vi "esm_Set Target CPU Monitoring__NATIONAL INSTRUMENTS.vi"(8 "error in (no error)":errorcluster, 10 "CPU Monitoring On":bool=TRUE, 11 "application reference":refnum<vi>) -> (0 "error out":errorcluster, 3 "application reference out":refnum<vi>)   [LabVIEW 2010, in "kevLib2010.lvlib"]
uses:
  kevLib2010.lvlib
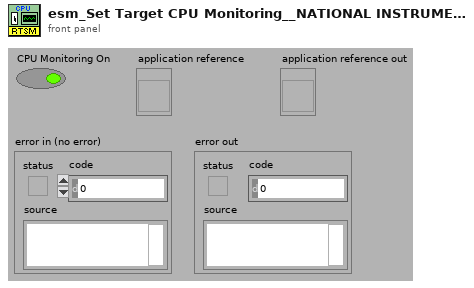
[diagram p1: front panel]
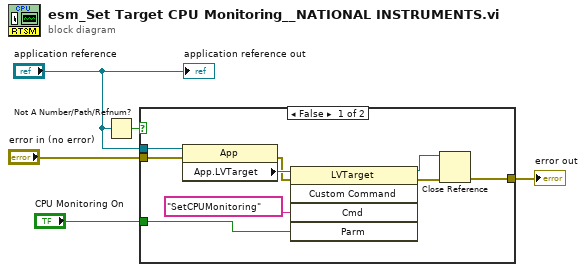
[diagram p0: block diagram]
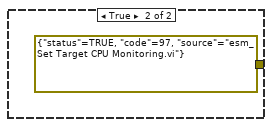
[diagram p2: hidden frame]
diagram:
  n1 = Not A Number/Path/Refnum?(number/path/refnum="application reference") -> (NaN/Path/Refnum?=w3:bool)
  n2 = case shown="False" w3 {
    tunnel: "error in (no error)" -> [w9 _]
    tunnel: "application reference" -> [w8 _]
    tunnel: [w7 errorcluster {"status"=TRUE, "code"=97, "source"="esm_Set Target CPU Monitoring.vi"} ("error out")] -> w4
    tunnel: "CPU Monitoring On" -> [w6 _]
    frame False {
      n3 = property class="App"(reference=w8, error in=w9) -> (error out=w12:errorcluster, "App.LVTarget"=w14:refnum<vi>)  [unwired: 1 out]
      n4 = invoke class="LVTarget" method="Custom Command"(reference=w14, error in=w12, "Cmd"="SetCPUMonitoring" ("CommandName"), "Parm"=w6) -> (reference out=w10:refnum<vi>, error out=w11:errorcluster)  [unwired: 1 in, 3 out]
      n5 = Close Reference(reference=w10, error in (no error)=w11) -> (error out=w7:errorcluster)
    }
    frame True {
    }
  }
  "error out" <- w4
  "application reference out" <- "application reference"
